vi "求组合(公式法）vi.vi"(1 "k":i32=100, 2 "n":i32=100) -> (0 "C(n,k)":dbl)   [LabVIEW 2012]
doc: "功能：\n\n利用组合公式求组合。\n\n公式：\n\nC(n,k)=n!/(k!*(n-k)!\n\n该VI存在下列两个重要的问题，将在其它组合VI中改进：\n1、当阶乘给定超过170时导致阶乘为无穷大，因此限制了计算范围。\n2、直接使用公式导致了大量的重复计算，效率极低。\n\nCSXCS_366创建"
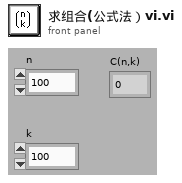
[diagram p1: front panel]
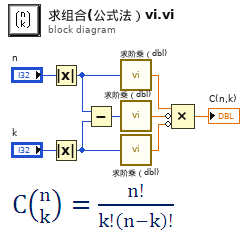
[diagram p0: block diagram]
diagram:
  n1 = Absolute Value(x="n") -> (abs(x)=w7:i32)
  n2 = Absolute Value(x="k") -> (abs(x)=w6:i32)
  n3 = Subtract(x=w7, y=w6) -> (x-y=w5:i32)
  n4 = call "求阶乘（dbl).vi"("Num"=w7) -> ("Fract"=w4:dbl)
  n5 = call "求阶乘（dbl).vi"("Num"=w5) -> ("Fract"=w2:dbl)
  n6 = call "求阶乘（dbl).vi"("Num"=w6) -> ("Fract"=w1:dbl)
  n7 = Compound Arithmetic op=MULTIPLY(w4, invert w2, invert w1) -> (→"C(n,k)":dbl)
